vi "ProdaNG.File.ExportToDB.vi"(5 "Identification":T1, 6 "reason":string, 7 "TestStepsTree":refnum<vi>, 8 "error in (no error)":errorcluster, 10 "FileContent":T2, 11 "dbHandleIn":i32) -> (0 "error out":errorcluster, 3 "dbHandle":i32)   [LabVIEW 2016]
uses:
  ProdaNG.File.Sequence.ctl
  ProdaNG.Tree.Fglb.Value.ctl
  ProdaNG.File.Step.ctl
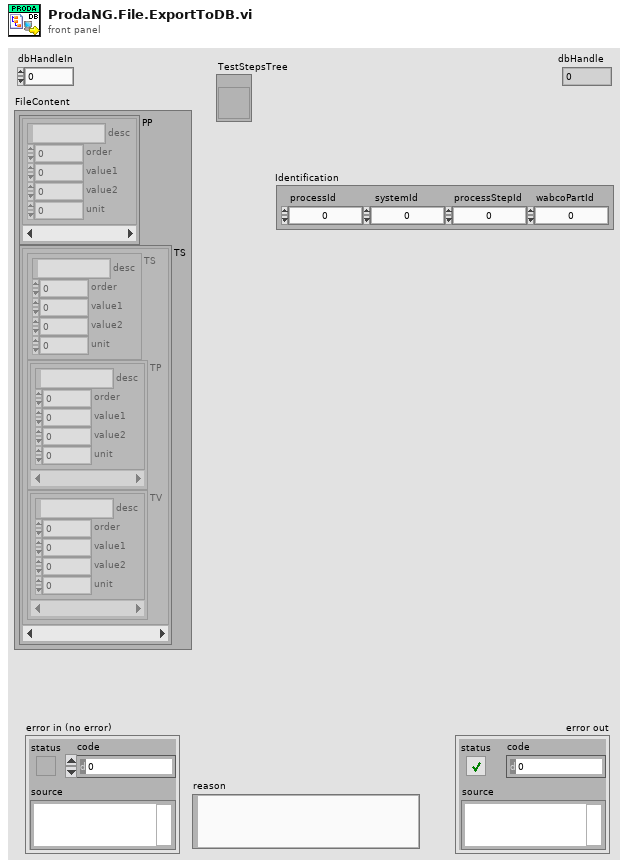
[diagram p1: front panel]
types:
  T1 = cluster{"processId":i32, "systemId":i32, "processStepId":i32, "wabcoPartId":i32}
  T2 = typedef "ProdaNG.File.Sequence.ctl" = cluster{"PP":T3[], "TS":T4[]}
  T3 = typedef "ProdaNG.Tree.Fglb.Value.ctl" = cluster{"desc":string, "order":i32, "value1":dbl, "value2":dbl, "unit":i32}
  T4 = typedef "ProdaNG.File.Step.ctl" = cluster{"TS":T3, "TP":T3[], "TV":T3[]}
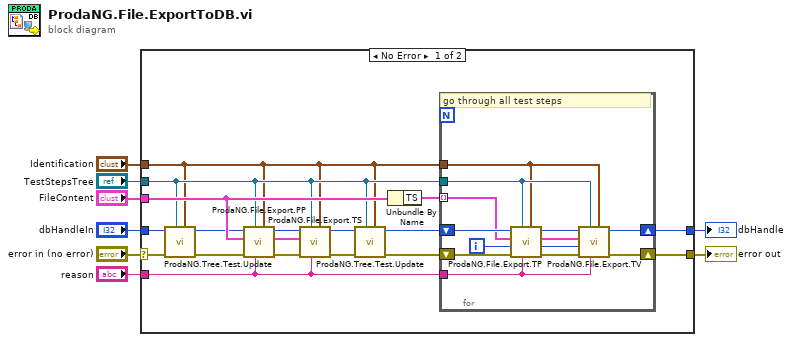
[diagram p0: block diagram]
diagram:
  n1 = case shown="No Error" "error in (no error)" {
    selector: "error in (no error)" -> [w19 w38]
    tunnel: [w24 w38] -> w8
    tunnel: "dbHandleIn" -> [w18 w37]
    tunnel: [w25 w37] -> w5
    tunnel: "FileContent" -> [w20 _]
    tunnel: "reason" -> [w9 _]
    tunnel: "Identification" -> [w10 _]
    tunnel: "TestStepsTree" -> [w14 _]
    frame No Error {
      n2 = call "ProdaNG.Tree.Test.Update.vi"("Identification"=w10, "TreeControl in"=w14, "error in (no error)"=w19, "dbHandle in"=w18) -> ("error out"=w17:errorcluster, "dbHandle out"=w16:i32)  [unwired: 4 in, 2 out]
      n3 = call "ProdaNG.File.Export.PP.vi"("Identification"=w10, "reason"=w9, "TestStepsTree"=w14, "error in (no error)"=w17, "FileContent"=w20, "dbHandleIn"=w16) -> ("error out"=w21:errorcluster, "dbHandle"=w22:i32)  [unwired: 4 in]
      n4 = call "ProdaNG.File.Export.TS.vi"("Identification"=w10, "reason"=w9, "TestStepsTree"=w14, "error in (no error)"=w21, "FileContent"=w20, "dbHandleIn"=w22) -> ("error out"=w13:errorcluster, "dbHandle"=w15:i32)  [unwired: 4 in]
      n5 = call "ProdaNG.Tree.Test.Update.vi"("Identification"=w10, "TreeControl in"=w14, "error in (no error)"=w13, "dbHandle in"=w15) -> ("error out"=w11:errorcluster, "dbHandle out"=w12:i32)  [unwired: 4 in, 2 out]
      n6 = Unbundle By Name(w20) -> ("TS"=w23:T4[])
      n7 = for {
        shift-right: [w32] -> w25
        shift-left: w12 -> [w36]
        shift-right: [w33] -> w24
        shift-left: w11 -> [w31]
        tunnel: w10 -> [w28]
        tunnel: w14 -> [w29]
        tunnel: w23 -> [w27] mode=indexing
        tunnel: w9 -> [w30]
        i -> [w26]
        # "go through all test steps"
        n8 = call "ProdaNG.File.Export.TP.vi"("Identification"=w28, "reason"=w30, "TestStepsTree"=w29, "error in (no error)"=w31, "Idx"=w26, "TS"=w27, "dbHandleIn"=w36) -> ("error out"=w35:errorcluster, "dbHandle"=w34:i32)  [unwired: 3 in]
        n9 = call "ProdaNG.File.Export.TV.vi"("Identification"=w28, "reason"=w30, "TestStepsTree"=w29, "error in (no error)"=w35, "Idx"=w26, "TS"=w27, "dbHandleIn"=w34) -> ("error out"=w33:errorcluster, "dbHandle"=w32:i32)  [unwired: 3 in]
      }
    }
    frame Error {
    }
  }
  "error out" <- w8
  "dbHandle" <- w5
